vi "calcu extrana.vi"() -> ()   [LabVIEW 2020]
panel:
  out "Negativo \n VALOR 1":bool
  out "Negativo \n VALOR 2":bool
  in  "Ring":u16(ring) items=["SOLO VALOR 1", "OP. CON LOS 2 VALORES", "SOLO VALOR 2"]
  in  "VALOR 1":dbl
  in  "VALOR 2":dbl
  in  "Enum":T1(ring) caption="OP BASICAS"
  in  "stop":bool
  out "Respuesta":dbl
  in  "Op.Complejas":T2(ring)
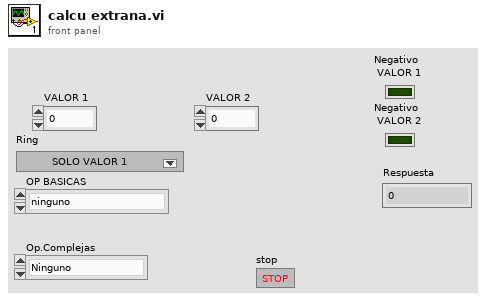
[diagram p1: front panel]
types:
  T1 = enum16{"ninguno", "suma", "resta", "multiplicacion", "division", "Elevar V2 a la V1", "Elevar V1 a la V2"}
  T2 = enum16{"Ninguno", "Raiz Cuadrada", "Pot. Cuadrada", "SEN", "COS", "TAN", "º --> RAD"}
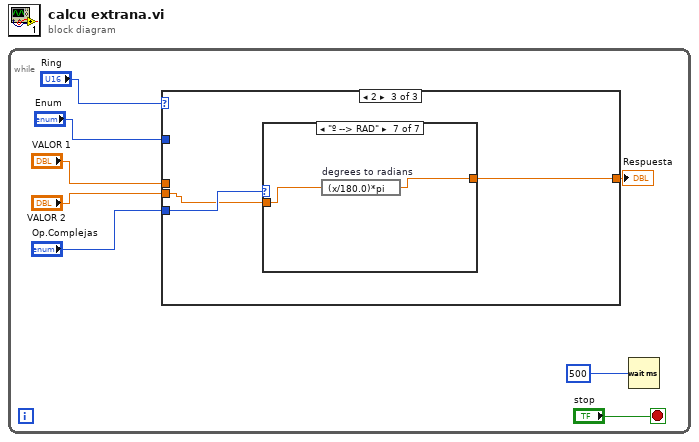
[diagram p0: block diagram]
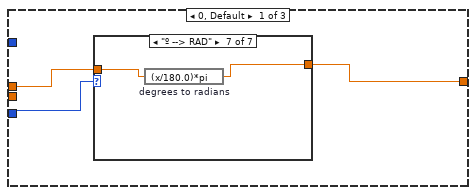
[diagram p2: hidden frame]
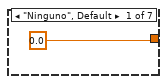
[diagram p3: hidden frame]
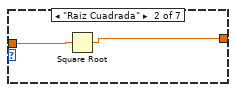
[diagram p4: hidden frame]
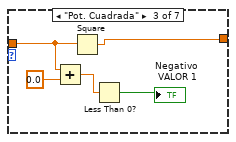
[diagram p5: hidden frame]
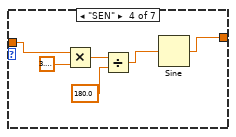
[diagram p6: hidden frame]
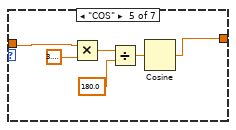
[diagram p7: hidden frame]
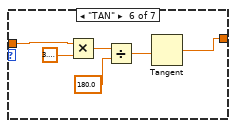
[diagram p8: hidden frame]
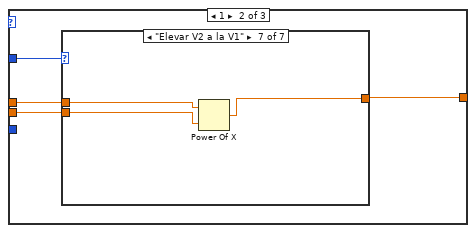
[diagram p9: hidden frame]
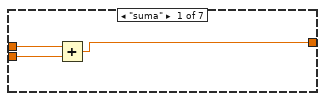
[diagram p10: hidden frame]
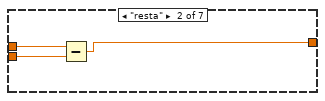
[diagram p11: hidden frame]
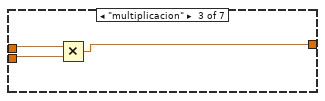
[diagram p12: hidden frame]
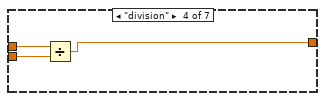
[diagram p13: hidden frame]
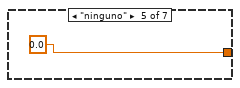
[diagram p14: hidden frame]
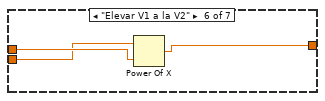
[diagram p15: hidden frame]
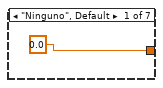
[diagram p16: hidden frame]
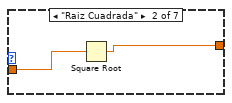
[diagram p17: hidden frame]
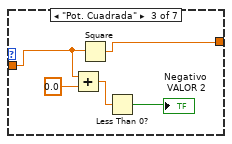
[diagram p18: hidden frame]
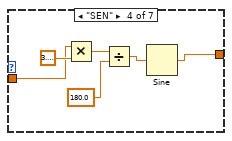
[diagram p19: hidden frame]
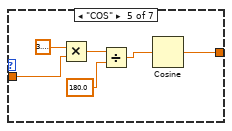
[diagram p20: hidden frame]
diagram:
  n1 = while {
    stop <- "stop" stop-if-true
    n2 = case shown="2" "Ring" {
      tunnel: "VALOR 1" -> [w11 w43 _]
      tunnel: "VALOR 2" -> [_ w42 w63]
      tunnel: [w10 w41 w64] -> w5
      tunnel: "Enum" -> [_ w40 _]
      tunnel: "Op.Complejas" -> [w9 _ w65]
      frame 0, Default {
        n3 = case shown="\"º --> RAD\"" w9 {
          tunnel: w11 -> [_ w14 w18 w24 w27 w33 w39]
          tunnel: [0.0 w13 w19 w25 w31 w37 w38] -> w10
          frame "Ninguno", Default {
          }
          frame "Raiz Cuadrada" {
            n4 = Square Root(x=w14) -> (sqrt(x)=w13:dbl)
          }
          frame "Pot. Cuadrada" {
            n5 = Add(x=w18, y=0.0) -> (x+y=w15:dbl)
            n6 = Square(x=w18) -> (x^2=w19:dbl)
            n7 = Less Than 0?(x=w15) -> (x < 0?=→"Negativo \n VALOR 1":bool)
          }
          frame "SEN" {
            n8 = Multiply(x=w24, y=3.141592653589793) -> (x*y=w22:dbl)
            n9 = Divide(x=w22, y=180.0) -> (x/y=w20:dbl)
            n10 = Sine(x=w20) -> (sin(x)=w25:dbl)
          }
          frame "COS" {
            n11 = Multiply(x=w27, y=3.141592653589793) -> (x*y=w29:dbl)
            n12 = Divide(x=w29, y=180.0) -> (x/y=w26:dbl)
            n13 = Cosine(x=w26) -> (cos(x)=w31:dbl)
          }
          frame "TAN" {
            n14 = Multiply(x=w33, y=3.141592653589793) -> (x*y=w35:dbl)
            n15 = Divide(x=w35, y=180.0) -> (x/y=w32:dbl)
            n16 = Tangent(1:w32) -> (0:w37:dbl)
          }
          frame "º --> RAD" {
            n17 = expression code="(x/180.0)*pi" "degrees to radians"(w39) -> (w38:dbl)
          }
        }
      }
      frame 1 {
        n18 = case shown="\"Elevar V2 a la V1\"" w40 {
          tunnel: w43 -> [w46 w49 w52 w55 _ w59 w61]
          tunnel: w42 -> [w45 w48 w51 w54 _ w58 w62]
          tunnel: [w44 w47 w50 w53 0.0 w57 w60] -> w41
          frame "suma" {
            n19 = Add(x=w46, y=w45) -> (x+y=w44:dbl)
          }
          frame "resta" {
            n20 = Subtract(x=w49, y=w48) -> (x-y=w47:dbl)
          }
          frame "multiplicacion" {
            n21 = Multiply(x=w52, y=w51) -> (x*y=w50:dbl)
          }
          frame "division" {
            n22 = Divide(x=w55, y=w54) -> (x/y=w53:dbl)
          }
          frame "ninguno" {
          }
          frame "Elevar V1 a la V2" {
            n23 = Power Of X(1:w59, 2:w58) -> (0:w57:dbl)
          }
          frame "Elevar V2 a la V1" {
            n24 = Power Of X(1:w62, 2:w61) -> (0:w60:dbl)
          }
        }
      }
      frame 2 {
        n25 = case shown="\"º --> RAD\"" w65 {
          tunnel: [0.0 w68 w73 w74 w80 w86 w92] -> w64
          tunnel: w63 -> [_ w67 w71 w76 w84 w88 w93]
          frame "Ninguno", Default {
          }
          frame "Raiz Cuadrada" {
            n26 = Square Root(x=w67) -> (sqrt(x)=w68:dbl)
          }
          frame "Pot. Cuadrada" {
            n27 = Add(x=w71, y=0.0) -> (x+y=w70:dbl)
            n28 = Square(x=w71) -> (x^2=w73:dbl)
            n29 = Less Than 0?(x=w70) -> (x < 0?=→"Negativo \n VALOR 2":bool)
          }
          frame "SEN" {
            n30 = Multiply(x=w76, y=3.141592653589793) -> (x*y=w78:dbl)
            n31 = Divide(x=w78, y=180.0) -> (x/y=w75:dbl)
            n32 = Sine(x=w75) -> (sin(x)=w74:dbl)
          }
          frame "COS" {
            n33 = Multiply(x=3.141592653589793, y=w84) -> (x*y=w83:dbl)
            n34 = Divide(x=w83, y=180.0) -> (x/y=w81:dbl)
            n35 = Cosine(x=w81) -> (cos(x)=w80:dbl)
          }
          frame "TAN" {
            n36 = Multiply(x=3.141592653589793, y=w88) -> (x*y=w90:dbl)
            n37 = Divide(x=w90, y=180.0) -> (x/y=w87:dbl)
            n38 = Tangent(1:w87) -> (0:w86:dbl)
          }
          frame "º --> RAD" {
            n39 = expression code="(x/180.0)*pi" "degrees to radians"(w93) -> (w92:dbl)
          }
        }
      }
    }
    "Respuesta" <- w5
    n40 = Wait (ms)(milliseconds to wait=u32 500) -> ()  [unwired: 1 out]
  }
